vi "Tosca-Initialize AI.vi"(0 "AI":T1, 9 "T (ms)":dbl=500.0 caption="Frame size (ms)", 11 "error in (no error)":errorcluster) -> (15 "error out":errorcluster)   [LabVIEW 2020]
uses:
  Typedefs/Tosca-AI.ctl
  epl-vi-lib/PXI DAQ VIs/AIDI/Typedefs/AIDI-Config.ctl
  epl-vi-lib/PXI DAQ VIs/AIDI/Typedefs/AIDI-Output Spec.ctl
  epl-vi-lib/PXI DAQ VIs/AIDI/Typedefs/DI-Output Spec.ctl
  epl-vi-lib/Connection VIs/Type Defs/CM-IO Type.ctl
  epl-vi-lib/PXI DAQ VIs/AIDI/Typedefs/AIDI-Action.ctl
  Sub VIs/Tosca-Globals.vi
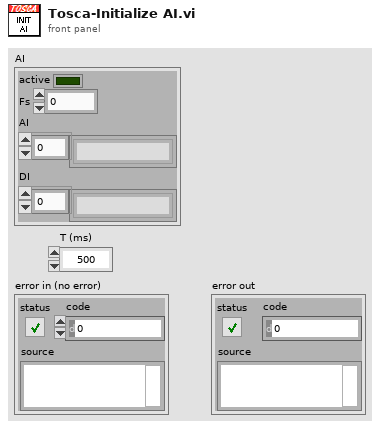
[diagram p1: front panel]
types:
  T1 = typedef "Tosca-AI.ctl" = cluster{"active":bool, "Fs":dbl, "AI":string[], "DI":string[]}
  T2 = typedef "AIDI-Action.ctl" = enum16{"Configure", "Initialize", "Start", "Read", "Clean up", "Init & Start", "Config & Test", "Position"}
  T3 = typedef "CM-IO Type.ctl" = enum16{"Analog Outputs", "Analog Inputs", "Digital Outputs", "Digital Inputs"}
  T4 = typedef "AIDI-Config.ctl" = cluster{"AI":T5, "DI":T6, "ExtTrig":bool}
  T5 = typedef "AIDI-Output Spec.ctl" = cluster{"Channels":string[], "Fs (Hz)":dbl, "Npts":i32}
  T6 = typedef "DI-Output Spec.ctl" = cluster{"Channels":string[], "Fs (Hz)":dbl, "Npts":i32, "Port":string}
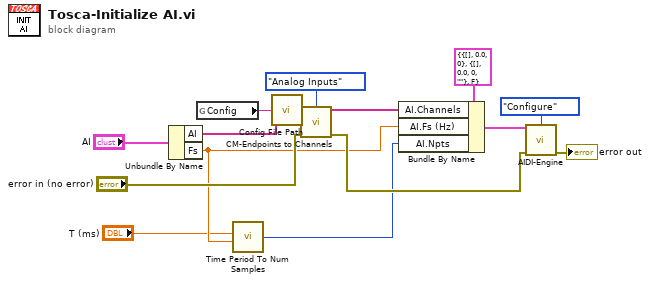
[diagram p0: block diagram]
diagram:
  n1 = Unbundle By Name("AI") -> ("AI"=w12:string[], "Fs"=w4:dbl)
  n2 = global read "Tosca-Globals.vi" "Config"() -> (w1:string)
  n3 = call "Time Period To Num Samples.vi"("Duration (ms)"="T (ms)", "Sampling rate (Hz)"=w4) -> ("Samples"=w2:i32)  [unwired: 5 in]
  n4 = call "Config File Path.vi"("AppName"=w1) -> ("Default config file name"=w15:path)
  n5 = call "CM-Endpoints to Channels.vi"("Path"=w15, "IO Type"=CM-IO_Type."Analog Inputs", "Requested Endpoints"=w12, "error in (no error)"="error in (no error)") -> ("IO Channels"=w10:string[], "error out"=w6:errorcluster)  [unwired: 10 in]
  n6 = Bundle By Name(cluster=T4 {"AI"={"Channels"=[], "Fs (Hz)"=0.0, "Npts"=0}, "DI"={"Channels"=[], "Fs (Hz)"=0.0, "Npts"=0, "Port"=""}, "ExtTrig"=FALSE} ("Config"), "AI.Channels"=w10, "AI.Fs (Hz)"=w4, "AI.Npts"=w2) -> (w9:T4)
  n7 = call "AIDI-Engine.vi"("Config"=w9, "Action"=AIDI-Action."Configure", "error in (no error)"=w6) -> ("error out"=→"error out":errorcluster)  [unwired: 9 in, 3 out]
